vi "Initialize.vi"(0 "Transaction in":refnum<class "Transaction.lvclass">, 1 "Reference":string, 5 "Date":timestamp, 7 "Amount":dbl, 9 "Description":string, 11 "error in (no error)":errorcluster, 12 "Category":string) -> (4 "Transaction out":refnum<class "Transaction.lvclass">, 15 "error out":errorcluster)   [LabVIEW 2018, in "Transaction.lvclass"]
uses:
  Transaction.lvclass
  Transaction.lvclass/Transaction.ctl
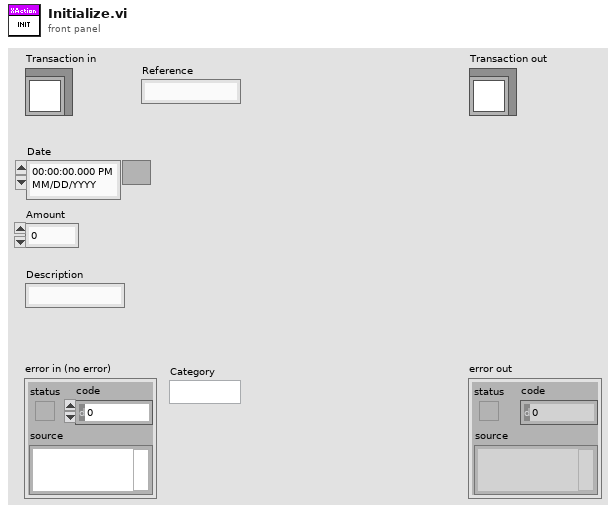
[diagram p1: front panel]
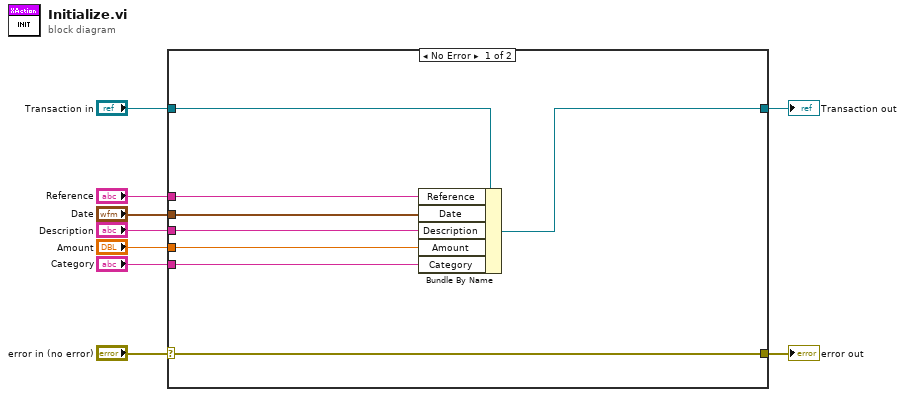
[diagram p0: block diagram]
diagram:
  n1 = case shown="No Error" "error in (no error)" {
    selector: "error in (no error)" -> [w17 w19]
    tunnel: [w17 w19] -> w8
    tunnel: [w15 w18] -> w6
    tunnel: "Transaction in" -> [w16 w18]
    tunnel: "Reference" -> [w14 _]
    tunnel: "Date" -> [w13 _]
    tunnel: "Description" -> [w12 _]
    tunnel: "Amount" -> [w11 _]
    tunnel: "Category" -> [w10 _]
    frame No Error {
      n2 = Bundle By Name(cluster=w16, "Reference"=w14, "Date"=w13, "Description"=w12, "Amount"=w11, "Category"=w10) -> (w15:refnum<class "Transaction.lvclass">)
    }
    frame Error {
    }
  }
  "error out" <- w8
  "Transaction out" <- w6
